vi "writeAttributesToFile_action.vi"(0 "HGF_ImaqDx":refnum<class "HGF_ImaqDx.lvclass">, 2 "Filename":path, 5 "error in (no error)":errorcluster) -> (14 "dup HGF_ImaqDx":refnum<class "HGF_ImaqDx.lvclass">, 19 "error out":errorcluster)   [LabVIEW 2014, in "HGF_IMAQ.lvlib" / "HGF_ImaqDx.lvclass"]
doc: "Saves a configuration file for a camera."
uses:
  HGF_ImaqDx.lvclass
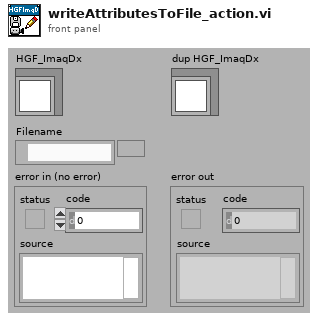
[diagram p1: front panel]
types:
  T1 = typedef "IMAQdx.ctl" = refnum<k21>
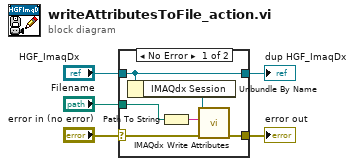
[diagram p0: block diagram]
diagram:
  n1 = case shown="No Error" "error in (no error)" {
    selector: "error in (no error)" -> [w11 w12]
    tunnel: [w6 w13] -> w4
    tunnel: "HGF_ImaqDx" -> [w6 w13]
    tunnel: [w10 w12] -> w2
    tunnel: "Filename" -> [w8 _]
    frame No Error {
      n2 = Unbundle By Name(w6) -> ("IMAQdx Session"=w7:T1)
      n3 = Path To String(path=w8) -> (string=w9:string)
      n4 = call <vilib>:"IMAQdx Write Attributes.vi"("error in"=w11, "Filename"=w9, "Session In"=w7) -> ("error out"=w10:errorcluster)  [unwired: 7 in, 1 out]
    }
    frame Error {
    }
  }
  "error out" <- w2
  "dup HGF_ImaqDx" <- w4
